vi "Create Signature Key v4.vi"(0 "AWS Service":string, 1 "Region":string, 2 "date/time string":string, 3 "Secret Key":string) -> (7 "Keyed-Hash":string)   [LabVIEW 2015, in "AWS Core.lvlib"]
uses:
  AWS Core.lvlib
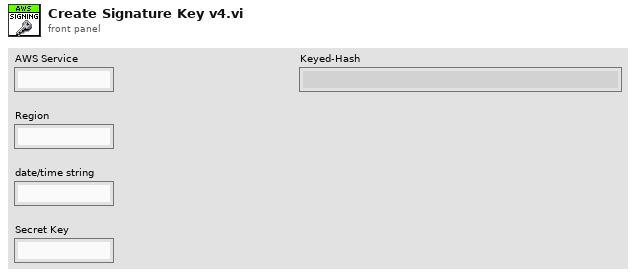
[diagram p1: front panel]
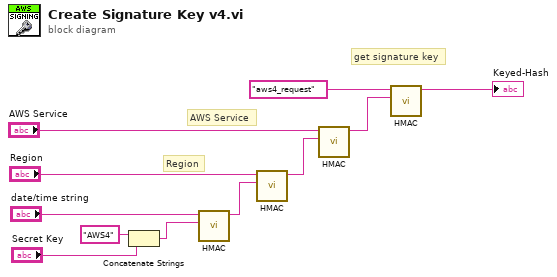
[diagram p0: block diagram]
diagram:
  # "AWS Service"
  # "Region"
  # "get signature key"
  n1 = Concatenate Strings("AWS4" ("string"), "Secret Key") -> (w4:string)
  n2 = call "HMAC.vi"("Key"=w4, "Message"="date/time string") -> ("Keyed Hash"=w3:string)  [unwired: 9 in]
  n3 = call "HMAC.vi"("Key"=w3, "Message"="Region") -> ("Keyed Hash"=w2:string)  [unwired: 9 in]
  n4 = call "HMAC.vi"("Key"=w2, "Message"="AWS Service") -> ("Keyed Hash"=w1:string)  [unwired: 9 in]
  n5 = call "HMAC.vi"("Key"=w1, "Message"="aws4_request") -> ("Keyed Hash"=→"Keyed-Hash":string)  [unwired: 9 in]
